vi "NetworkServerDiscovery.vi"() -> ()   [LabVIEW 2012, in "Phidget Common.lvlib"]
uses:
  <instrlib>/Phidgets/Phidget Common/Phidget Common.lvlib
  <instrlib>/Phidgets/Phidget Accelerometer/Public/AccelerometerStart.vi
  <instrlib>/Phidgets/Phidget Accelerometer/Public/AccelerometerClose.vi
  <instrlib>/Phidgets/Phidget Accelerometer/Phidget Accelerometer.lvlib
panel:
  out "Acceleration":dbl[](array[numeric])
  out "error out":errorcluster
  in  "Device Info":T1={"Serial Number"=-1, "Channel"=0, "Port"=0}
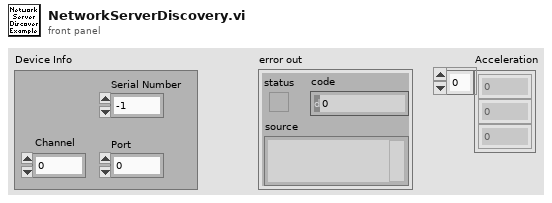
[diagram p1: front panel]
types:
  T1 = cluster{"Serial Number":i32, "Channel":i32, "Port":i32}
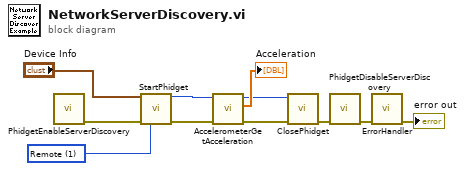
[diagram p0: block diagram]
diagram:
  w11 = u16 1 items=["No Preference", "Remote", "Local"] ("Connection")
  n1 = call <instrlib>:"PhidgetEnableServerDiscovery.vi"() -> ("error out"=w8:errorcluster)  [unwired: 11 in]
  n2 = call-poly <instrlib>:"StartPhidget.vi"("Device Info"="Device Info", "error in (no error)"=w8, "Connection"=w11) -> ("Phidget ID"=w4:u64, "error out"=w3:errorcluster)  [unwired: 9 in, 2 out]
  n3 = call <instrlib>:"AccelerometerGetAcceleration.vi"("error in (no error)"=w3, "Device In"=w4) -> ("error out"=w2:errorcluster, "Acceleration"=→"Acceleration":dbl[], "Device Out"=w1:u64)  [unwired: 6 in]
  n4 = call-poly <instrlib>:"ClosePhidget.vi"("error in"=w2, "Device In"=w1) -> ("error out"=w9:errorcluster)  [unwired: 9 in]
  n5 = call <instrlib>:"PhidgetDisableServerDiscovery.vi"("error in"=w9) -> ("error out"=w7:errorcluster)  [unwired: 10 in]
  n6 = call <instrlib>:"ErrorHandler.vi"("error in"=w7) -> ("error out"=→"error out":errorcluster)  [unwired: 9 in, 1 out]
